vi "LVIS_ReadConfigDB.vi"(8 "Error In":errorcluster) -> (0 "Error Out":errorcluster, 3 "Disable":bool)   [LabVIEW 2015]
doc: "Reads in the LVIS_Settings file configuration values and loads them to the appropiate variables."
uses:
  Globals/LVIS_DcGlobals.vi
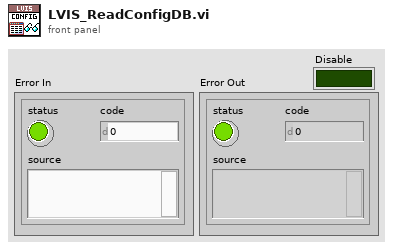
[diagram p1: front panel]
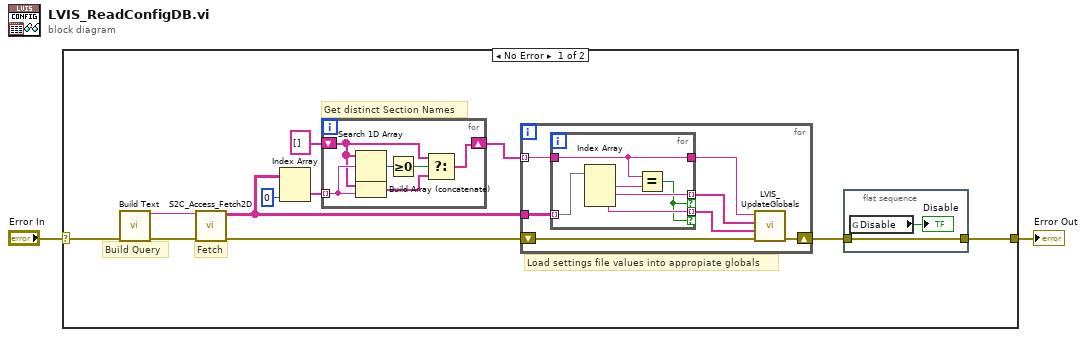
[diagram p0: block diagram]
diagram:
  n1 = case shown="No Error" "Error In" {
    selector: "Error In" -> [w5 w35]
    tunnel: [w3 w35] -> w1
    frame No Error {
      # "Load settings file values into appropiate globals"
      # "Get distinct Section Names"
      # "Fetch"
      # "Build Query"
      n2 = call "Build Text"("error in (no error)"=w5) -> ("Result"=w11:string, "error out"=w13:errorcluster)  [unwired: 13 in]
      n3 = call "S2C_Access_Fetch2D.vi"("Error In"=w13, "Query"=w11) -> ("Error Out"=w12:errorcluster, "Data"=w10:string[][])  [unwired: 8 in]
      n4 = Index Array(array=w10, index (col)=0 ("disabled index (col)")) -> (element=w8:string[])  [unwired: 1 in]
      n5 = for {
        shift-right: [w16] -> w6
        shift-left: string[] [] -> [w18]
        tunnel: w8 -> [w19] mode=indexing
        n6 = Search 1D Array(1D array=w18, element=w19) -> (index of element=w21:i32)  [unwired: 1 in]
        n7 = Build Array (concatenate)(w18, w19) -> (w17:string[])
        n8 = Greater Or Equal To 0?(x=w21) -> (x >= 0?=w20:bool)
        n9 = Select(t=w18, s=w20, f=w17) -> (s? t:f=w16:string[])
      }
      n10 = for {
        tunnel: w10 -> [w28]
        shift-right: [w26] -> w4
        shift-left: w12 -> [w27]
        tunnel: w6 -> [w23] mode=indexing
        n11 = for {
          tunnel: w28 -> [w34] mode=indexing
          tunnel: [w32] -> w25 mode=indexing if=w30
          tunnel: [w31] -> w24 mode=indexing if=w30
          tunnel: w23 -> [w29]
          tunnel: [w29] -> w22
          n12 = Index Array(array=w34) -> (element #1=w33:string, element #2=w32:string, element #3=w31:string)  [unwired: 3 in]
          n13 = Equal?(x=w29, y=w33) -> (x = y?=w30:bool)
        }
        n14 = call "LVIS_UpdateGlobals.vi"("Error In"=w27, "Values"=w24, "Keys"=w25, "Section"=w22) -> ("Error Out"=w26:errorcluster)  [unwired: 7 in]
      }
      n15 = flat-sequence {
        tunnel: w4 -> [w15]
        tunnel: [w15] -> w3
        frame #0 {
          n16 = global read "LVIS_DcGlobals.vi" "Disable"() -> (→"Disable":bool)
        }
      }
    }
    frame Error {
    }
  }
  "Error Out" <- w1
